vi "Generate.vi"(8 "error in (no error)":errorcluster, 9 "Message Queue":refnum<queue>, 10 "Advanced Waveform.lvclass In":refnum<class "Advanced Waveform.lvclass">, 11 "Generate in":refnum<class "Generate.lvclass">) -> (0 "error out":errorcluster, 1 "Message Queue Out":refnum<queue>, 2 "Advanced Waveform.lvclass Out":refnum<class "Advanced Waveform.lvclass">, 3 "Generate out":refnum<class "Generate.lvclass">)   [LabVIEW 2011, in "Generate.lvclass"]
uses:
  Generate.lvclass
  Advanced Waveform Class/Advanced Waveform.lvclass
  Message Class/Message.lvclass
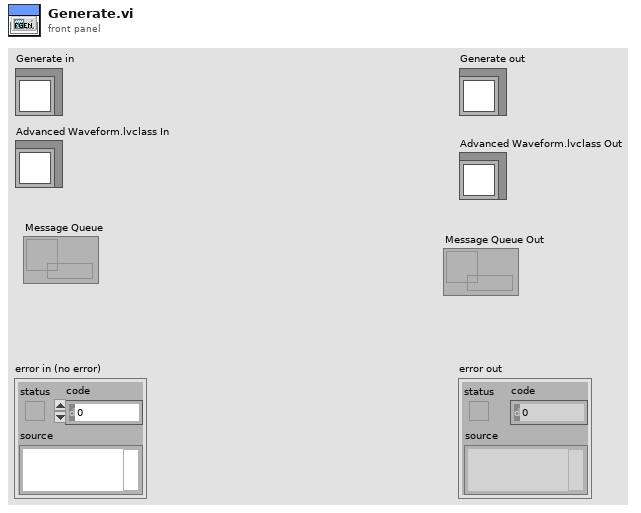
[diagram p1: front panel]
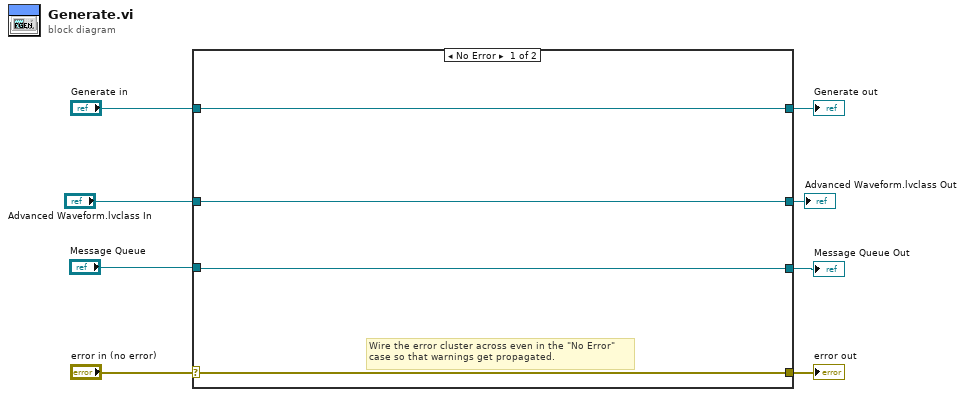
[diagram p0: block diagram]
diagram:
  n1 = case shown="No Error" "error in (no error)" {
    selector: "error in (no error)" -> [w11 w16]
    tunnel: [w11 w16] -> w7
    tunnel: [w12 w15] -> w5
    tunnel: "Generate in" -> [w12 w15]
    tunnel: "Advanced Waveform.lvclass In" -> [w10 w14]
    tunnel: [w10 w14] -> w3
    tunnel: "Message Queue" -> [w9 w13]
    tunnel: [w9 w13] -> w1
    frame No Error {
      # "Wire the error cluster across even in the \"No Error\"\ncase so that warnings get propagated."
    }
    frame Error {
    }
  }
  "error out" <- w7
  "Generate out" <- w5
  "Advanced Waveform.lvclass Out" <- w3
  "Message Queue Out" <- w1
